vi "Channel_ReadAndConvert.vi"(0 "Element In (2D Arr)":dbl[][](array[numeric]) format="%0.2f", 1 "Amplification (1E6) / V/A":dbl=1000000.0, 2 "Piezo Sensitivity (1.95) / nm V-1":dbl=1.95, 11 "Error in":errorcluster, 12 "Offset (0) / 1E-5 V":dbl, 13 "Piezo Amp (21.5)":dbl=21.5) -> (3 "Real Time Femto /V":dbl, 6 "Piezo / nm":dbl, 8 "Bias / V":dbl, 10 "G / G0":dbl, 15 "Error Out":errorcluster)   [LabVIEW 2025]
uses:
  <vilib>/Analysis/baseanly.llb/Mean (DBL).vi
  <vilib>/Analysis/NI_AALBase.lvlib
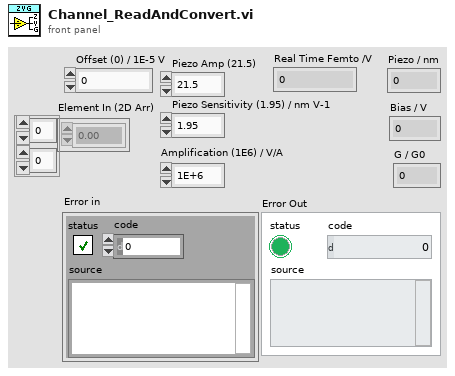
[diagram p1: front panel]
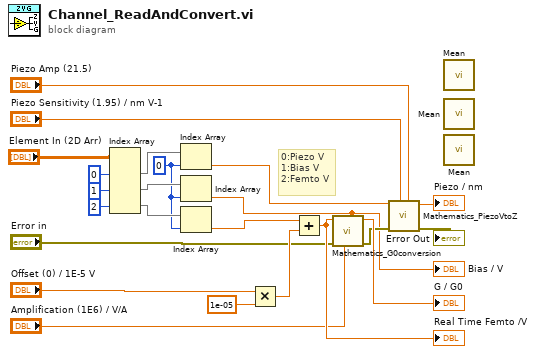
[diagram p0: block diagram]
diagram:
  w3 = 0 ("index")
  # "0:Piezo V\n1:Bias V\n2:Femto V"
  n1 = Index Array(array="Element In (2D Arr)", index (row) #1=0 ("index (row)"), index (row) #2=1 ("index (row)"), index (row) #3=2 ("index (row)")) -> (element #1=w7:dbl[], element #2=w5:dbl[], element #3=w4:dbl[])  [unwired: 3 in]
  n2 = Index Array(array=w7, index=w3) -> (element=w6:dbl)
  n3 = Index Array(array=w5, index=w3) -> (element=w2:dbl)
  "Bias / V" <- w2
  n4 = Index Array(array=w4, index=w3) -> (element=w1:dbl)
  n5 = Multiply(x="Offset (0) / 1E-5 V", y=1e-05) -> (x*y=w17:dbl)
  n6 = Add(x=w1, y=w17) -> (x+y=w18:dbl)
  "Real Time Femto /V" <- w18
  n7 = call "Mathematics_G0conversion.vi"("Bias (0.2) / V"=w2, "Amplification (1E6) / V/A"="Amplification (1E6) / V/A", "Error In"="Error in", "Femto Output (0) / V"=w18) -> ("Error Out"=w22:errorcluster, "G/G0"=→"G / G0":dbl)  [unwired: 6 in]
  n8 = call "Mathematics_PiezoVtoZ.vi"("Piezo Amp (21.5)"="Piezo Amp (21.5)", "Piezo Sensitivity (1.95) / nm V-1"="Piezo Sensitivity (1.95) / nm V-1", "Error In"=w22, "Piezo Signal In (0) / V"=w6) -> ("Error Out"=→"Error Out":errorcluster, "Piezo Signal Out / nm"=→"Piezo / nm":dbl)  [unwired: 6 in]
  n9 = call-poly <vilib>:"Mean.vi"() -> ()  [unwired: 1 in, 2 out]
  n10 = call-poly <vilib>:"Mean.vi"() -> ()  [unwired: 1 in, 2 out]
  n11 = call-poly <vilib>:"Mean.vi"() -> ()  [unwired: 1 in, 2 out]
